vi "Label Printing - Fail.vi"(3 "NGCODE":string, 4 "LINECODE":string, 5 "TIME":string, 6 "Print?":bool, 7 "PN":string, 8 "error in (no error)":errorcluster, 9 "SN":string, 10 "DT":string, 11 "Path":path=path "D:/Valeo/Micriphone Test/UI/ME79.btw") -> (0 "error out":errorcluster)   [LabVIEW 2018]
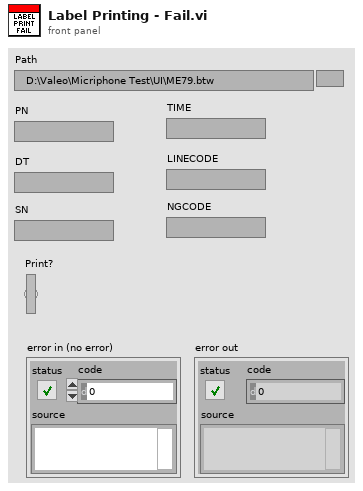
[diagram p1: front panel]
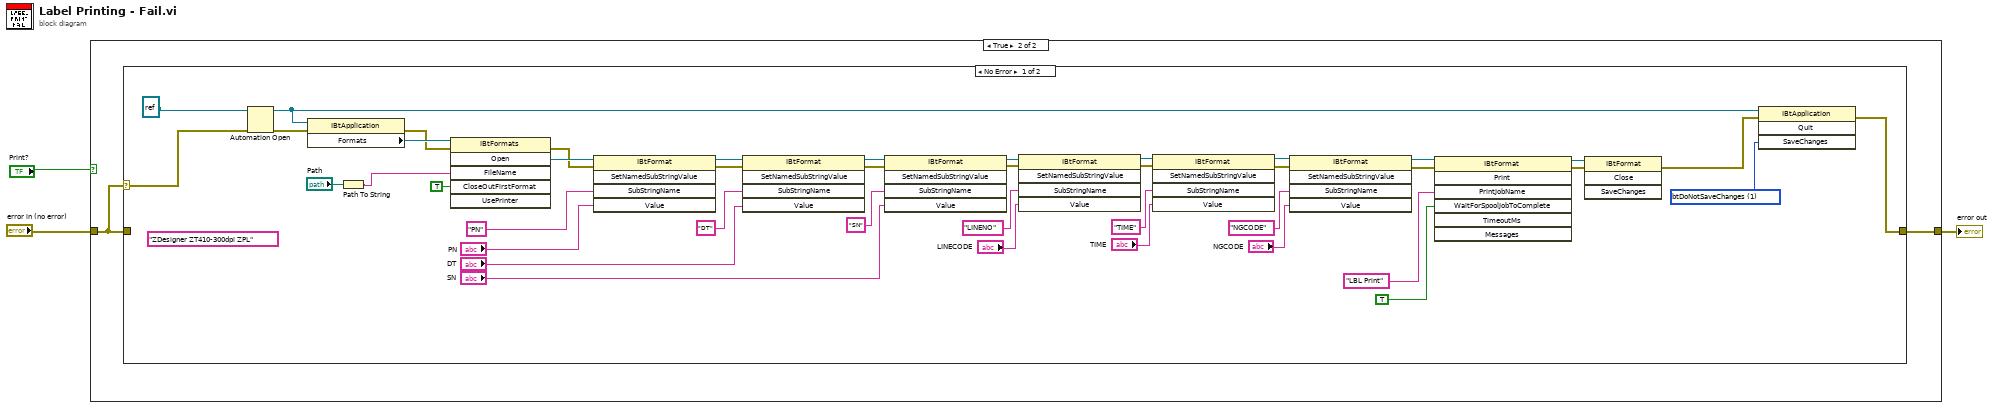
[diagram p0: block diagram]
diagram:
  n1 = case shown="True" "Print?" {
    tunnel: "error in (no error)" -> [w4 w5]
    tunnel: [w4 w6] -> w1
    frame False {
    }
    frame True {
      n2 = case shown="No Error" w5 {
        selector: w5 -> [w31 _]
        tunnel: [w32 w49] -> w6
        tunnel: w5 -> [_ w49]
        frame No Error {
          (unwired) "ZDesigner ZT410-300dpi ZPL" ("UsePrinter")
          w41 = 1 items=["btPromptSave", "btDoNotSaveChanges", "btSaveChanges"] ("SaveChanges")
          n3 = Automation Open(error in (no error)=w31, Automation Refnum=refnum<k7> refnum ("BarTender.IBtApplication")) -> (Automation Refnum=w42:refnum<k7>, error out=w48:errorcluster)  [unwired: 2 in]
          n4 = property class="IBtApplication"(reference=w42, error in=w48) -> (error out=w46:errorcluster, "Formats"=w47:refnum<k7>)  [unwired: 1 out]
          n5 = Path To String(path="Path") -> (string=w44:string)
          n6 = invoke class="IBtFormats" method="Open"(reference=w47, error in=w46, "FileName"=w44, "CloseOutFirstFormat"=TRUE) -> (error out=w38:errorcluster, "Open"=w39:refnum<k7>)  [unwired: 2 in, 4 out]
          n7 = invoke class="IBtFormat" method="SetNamedSubStringValue"(reference=w39, error in=w38, "SubStringName"="PN" ("FieldnameSampleDataList"), "Value"="PN") -> (reference out=w30:refnum<k7>, error out=w28:errorcluster)  [unwired: 1 in, 3 out]
          n8 = invoke class="IBtFormat" method="SetNamedSubStringValue"(reference=w30, error in=w28, "SubStringName"="DT" ("FieldnameSampleDataList"), "Value"="DT") -> (reference out=w29:refnum<k7>, error out=w27:errorcluster)  [unwired: 1 in, 3 out]
          n9 = invoke class="IBtFormat" method="SetNamedSubStringValue"(reference=w29, error in=w27, "SubStringName"="SN" ("FieldnameSampleDataList"), "Value"="SN") -> (reference out=w20:refnum<k7>, error out=w13:errorcluster)  [unwired: 1 in, 3 out]
          n10 = invoke class="IBtFormat" method="SetNamedSubStringValue"(reference=w20, error in=w13, "SubStringName"="LINENO" ("FieldnameSampleDataList"), "Value"="LINECODE") -> (reference out=w19:refnum<k7>, error out=w14:errorcluster)  [unwired: 1 in, 3 out]
          n11 = invoke class="IBtFormat" method="SetNamedSubStringValue"(reference=w19, error in=w14, "SubStringName"="TIME" ("FieldnameSampleDataList"), "Value"="TIME") -> (reference out=w18:refnum<k7>, error out=w15:errorcluster)  [unwired: 1 in, 3 out]
          n12 = invoke class="IBtFormat" method="SetNamedSubStringValue"(reference=w18, error in=w15, "SubStringName"="NGCODE" ("FieldnameSampleDataList"), "Value"="NGCODE") -> (reference out=w17:refnum<k7>, error out=w16:errorcluster)  [unwired: 1 in, 3 out]
          n13 = invoke class="IBtFormat" method="Print"(reference=w17, error in=w16, "PrintJobName"="LBL Print", "WaitForSpoolJobToComplete"=TRUE) -> (reference out=w37:refnum<k7>, error out=w36:errorcluster)  [unwired: 3 in, 5 out]
          n14 = invoke class="IBtFormat" method="Close"(reference=w37, error in=w36) -> (error out=w35:errorcluster)  [unwired: 2 in, 3 out]
          n15 = invoke class="IBtApplication" method="Quit"(reference=w42, error in=w35, "SaveChanges"=w41) -> (error out=w32:errorcluster)  [unwired: 1 in, 3 out]
        }
        frame Error {
        }
      }
    }
  }
  "error out" <- w1
